vi "Algorithm.vi"(4 "Algorithm Parameter":T2={"alpha Rbar"=1.0, "lambda w"=0.9, "lambda theta"=0.9, "alpha w"=0.1, "alpha theta"=0.01}, 6 "Basis":enum16{"Polynomial", "Fourier"}(ring), 8 "n":i32=1, 11 "Variable":T1={"state"=[0.0, 0.0, 0.0], "state'"=[0.0, 0.0, 0.0], "w"=[0.0], "zw"=[0.0], "theta"=[0.0], "ztheta"=[0.0], "R"=0.0, "Rbar"=0.0, "eligibility vector"=[0.0]} {"Rbar" format="%#_6f"; "R" format="%#_6f"}) -> (3 "Variable":T1)   [LabVIEW 2017]
uses:
  <vilib>/Analysis/baseanly.llb/Real Dot Product.vi
  <vilib>/Analysis/NI_AALBase.lvlib
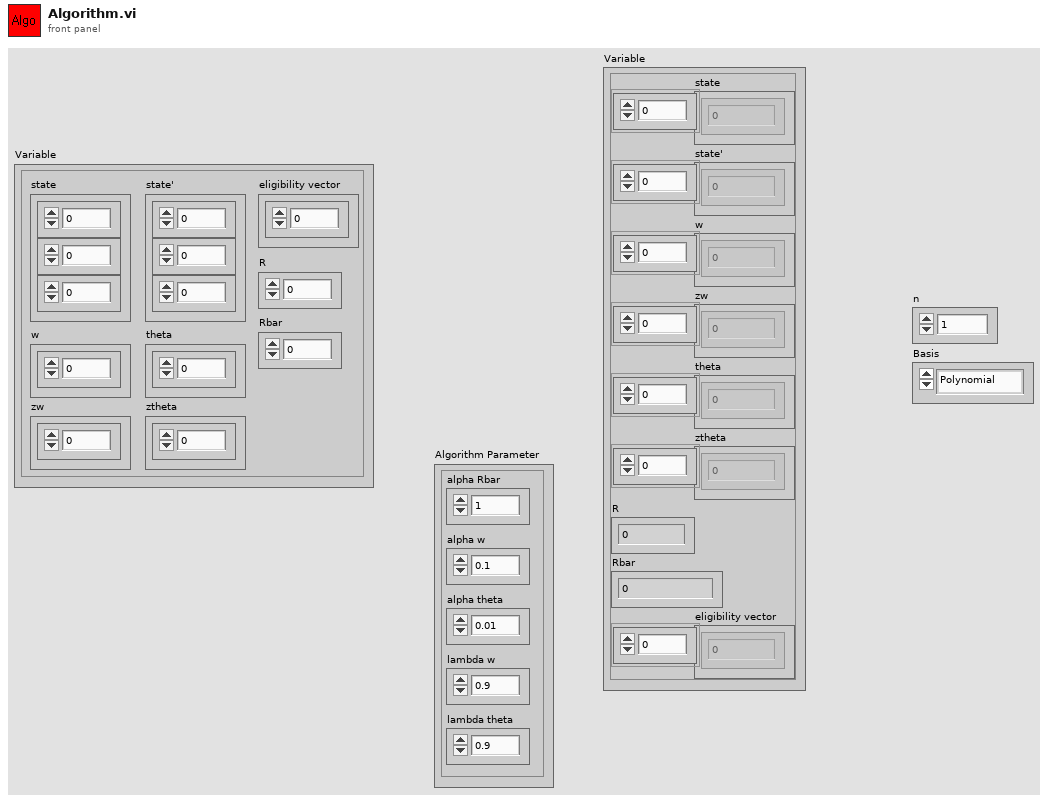
[diagram p1: front panel]
types:
  T1 = cluster{"state":dbl[], "state'":dbl[], "w":dbl[], "zw":dbl[], "theta":dbl[], "ztheta":dbl[], "R":dbl, "Rbar":dbl, "eligibility vector":dbl[]}
  T2 = cluster{"alpha Rbar":dbl, "lambda w":dbl, "lambda theta":dbl, "alpha w":dbl, "alpha theta":dbl}
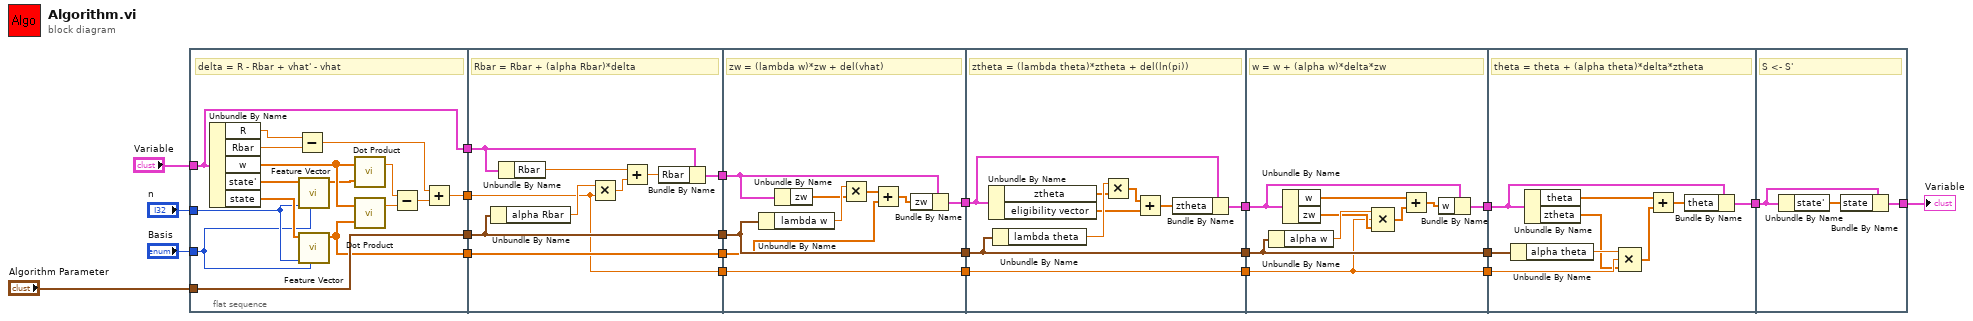
[diagram p0: block diagram]
diagram:
  n1 = flat-sequence {
    tunnel: "Variable" -> [w25]
    tunnel: "Algorithm Parameter" -> [w32]
    tunnel: [w32] -> w23
    tunnel: "n" -> [w28]
    tunnel: "Basis" -> [w27]
    tunnel: [w26] -> w9
    tunnel: [w25] -> w8
    tunnel: [w24] -> w6
    tunnel: [w45] -> w22
    tunnel: w23 -> [w43]
    tunnel: [w43] -> w21
    tunnel: w9 -> [w40]
    tunnel: w8 -> [w42]
    tunnel: [w41] -> w7
    tunnel: w6 -> [w41]
    tunnel: [w40] -> w5
    tunnel: w22 -> [w56]
    tunnel: [w54] -> w20
    tunnel: w21 -> [w52]
    tunnel: [w52] -> w19
    tunnel: w7 -> [w50]
    tunnel: w5 -> [w49]
    tunnel: [w49] -> w4
    tunnel: w20 -> [w65]
    tunnel: [w63] -> w18
    tunnel: w19 -> [w61]
    tunnel: [w61] -> w17
    tunnel: w4 -> [w58]
    tunnel: [w58] -> w3
    tunnel: w18 -> [w74]
    tunnel: [w73] -> w16
    tunnel: w17 -> [w71]
    tunnel: [w71] -> w15
    tunnel: w3 -> [w67]
    tunnel: [w67] -> w2
    tunnel: w16 -> [w83]
    tunnel: [w82] -> w14
    tunnel: w15 -> [w81]
    tunnel: w2 -> [w78]
    tunnel: [w85] -> w1
    tunnel: w14 -> [w87]
    frame #0 {
      # "delta = R - Rbar + vhat' - vhat"
      n2 = Unbundle By Name(w25) -> ("R"=w39:dbl, "Rbar"=w38:dbl, "w"=w37:dbl[], "state'"=w31:dbl[], "state"=w29:dbl[])
      n3 = Subtract(x=w39, y=w38) -> (x-y=w34:dbl)
      n4 = call "Feature Vector.vi"("Basis"=w27, "n"=w28, "input"=w31) -> ("feature vector"=w30:dbl[])  [unwired: 8 in]
      n5 = call "Feature Vector.vi"("Basis"=w27, "n"=w28, "input"=w29) -> ("feature vector"=w24:dbl[])  [unwired: 8 in]
      n6 = call-poly <vilib>:"Dot Product.vi"("Y Vector"=w30, "X Vector"=w37) -> ("X * Y"=w36:dbl)  [unwired: 1 out]
      n7 = call-poly <vilib>:"Dot Product.vi"("Y Vector"=w24, "X Vector"=w37) -> ("X * Y"=w35:dbl)  [unwired: 1 out]
      n8 = Subtract(x=w36, y=w35) -> (x-y=w33:dbl)
      n9 = Add(x=w34, y=w33) -> (x+y=w26:dbl)
    }
    frame #1 {
      # "Rbar = Rbar + (alpha Rbar)*delta"
      n10 = Unbundle By Name(w43) -> ("alpha Rbar"=w44:dbl)
      n11 = Unbundle By Name(w42) -> ("Rbar"=w48:dbl)
      n12 = Multiply(x=w44, y=w40) -> (x*y=w47:dbl)
      n13 = Add(x=w48, y=w47) -> (x+y=w46:dbl)
      n14 = Bundle By Name(cluster=w42, "Rbar"=w46) -> (w45:T1)
    }
    frame #2 {
      # "zw = (lambda w)*zw + del(vhat)"
      n15 = Unbundle By Name(w52) -> ("lambda w"=w53:dbl)
      n16 = Unbundle By Name(w56) -> ("zw"=w51:dbl[])
      n17 = Multiply(x=w53, y=w51) -> (x*y=w57:dbl[])
      n18 = Add(x=w57, y=w50) -> (x+y=w55:dbl[])
      n19 = Bundle By Name(cluster=w56, "zw"=w55) -> (w54:T1)
    }
    frame #3 {
      # "ztheta = (lambda theta)*ztheta + del(ln(pi))"
      n20 = Unbundle By Name(w65) -> ("ztheta"=w60:dbl[], "eligibility vector"=w59:dbl[])
      n21 = Unbundle By Name(w61) -> ("lambda theta"=w62:dbl)
      n22 = Multiply(x=w62, y=w60) -> (x*y=w66:dbl[])
      n23 = Add(x=w66, y=w59) -> (x+y=w64:dbl[])
      n24 = Bundle By Name(cluster=w65, "ztheta"=w64) -> (w63:T1)
    }
    frame #4 {
      # "w = w + (alpha w)*delta*zw"
      n25 = Unbundle By Name(w71) -> ("alpha w"=w72:dbl)
      n26 = Unbundle By Name(w74) -> ("w"=w70:dbl[], "zw"=w69:dbl[])
      n27 = Compound Arithmetic op=MULTIPLY(w72, w67, w69) -> (w75:dbl[])
      n28 = Add(x=w70, y=w75) -> (x+y=w68:dbl[])
      n29 = Bundle By Name(cluster=w74, "w"=w68) -> (w73:T1)
    }
    frame #5 {
      # "theta = theta + (alpha theta)*delta*ztheta"
      n30 = Unbundle By Name(w81) -> ("alpha theta"=w80:dbl)
      n31 = Unbundle By Name(w83) -> ("theta"=w79:dbl[], "ztheta"=w77:dbl[])
      n32 = Compound Arithmetic op=MULTIPLY(w80, w78, w77) -> (w84:dbl[])
      n33 = Add(x=w79, y=w84) -> (x+y=w76:dbl[])
      n34 = Bundle By Name(cluster=w83, "theta"=w76) -> (w82:T1)
    }
    frame #6 {
      # "S <- S'"
      n35 = Unbundle By Name(w87) -> ("state'"=w86:dbl[])
      n36 = Bundle By Name(cluster=w87, "state"=w86) -> (w85:T1)
    }
  }
  "Variable" <- w1
